vi "Register Create Test Node View.vi"(11 "Message Enqueuer in":refnum<class "Message Enqueuer.lvclass">) -> (3 "Message Enqueuer out":refnum<class "Message Enqueuer.lvclass">)   [LabVIEW 2013]
uses:
  <vilib>/ActorFramework/Message Enqueuer/Message Enqueuer.lvclass
  <vilib>/ActorFrameworkMVC/View Observer/Registration Message/Registration Message.lvclass
  <vilib>/ActorFrameworkMVC/View Observer/Data Message/Data Message.lvclass
  Models/Create Test Node Model Messages/Register Initialize Create Test Node Msg/Register Initialize Create Test Node Msg.lvclass
  Models/Create Test Node Model Messages/Register Set Create Test Node Key Focus Msg/Register Set Create Test Node Key Focus Msg.lvclass
  Views/Create Test Node View Messages/Conceret Initialize Create Test Node Msg/Conceret Initialize Create Test Node Msg.lvclass
  Views/Create Test Node View Messages/Conceret Set Create Test Node Key Focus Msg/Conceret Set Create Test Node Key Focus Msg.lvclass
  Views/Create Test Node View Messages/Conceret Create Test Node List Msg/Conceret Create Test Node List Msg.lvclass
  Models/Create Test Node Model Messages/Register Create Test Node List Msg/Register Create Test Node List Msg.lvclass
  <vilib>/ActorFrameworkMVC/UI Controller Messages/Subscribe View to Model Msg/Subscribe View to Model Msg.lvclass/Subscribe View to Model Msg.ctl
  <vilib>/ActorFramework/Message Enqueuer/Message Enqueuer.lvclass/Message Enqueuer.ctl
  <vilib>/ActorFramework/Message Enqueuer/Enqueue.vi
  <vilib>/ActorFramework/Message Priority Queue/Priority Enqueue.vi
  <vilib>/ActorFrameworkMVC/UI Controller Messages/Subscribe View to Model Msg/Subscribe View to Model Msg.lvclass
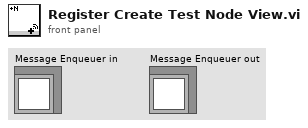
[diagram p1: front panel]
types:
  T1 = cluster{"Registration Message":string, "Data Message":string}[]
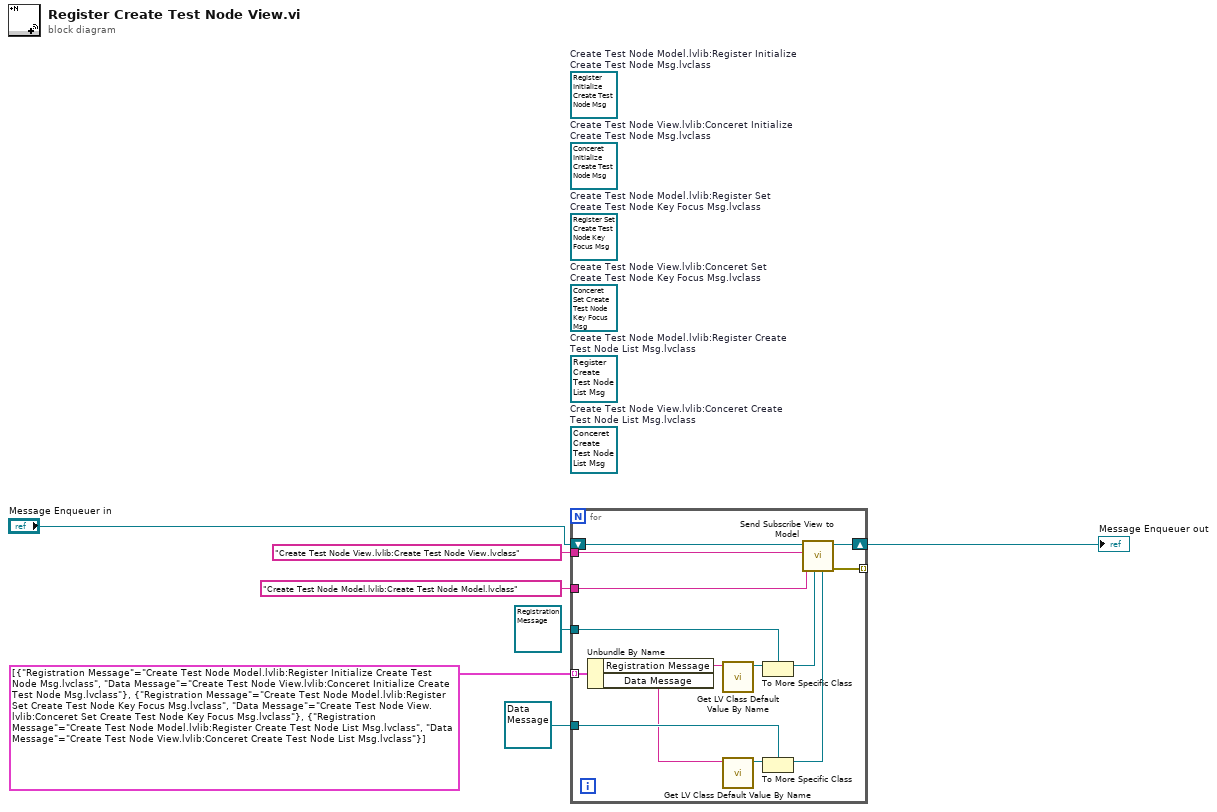
[diagram p0: block diagram]
diagram:
  (unwired) refnum<class "Register Create Test Node List Msg.lvclass"> refnum  # Create Test Node Model.lvlib:Register Create Test Node List Msg.lvclass
  (unwired) refnum<class "Conceret Create Test Node List Msg.lvclass"> refnum  # Create Test Node View.lvlib:Conceret Create Test Node List Msg.lvclass
  (unwired) refnum<class "Conceret Set Create Test Node Key Focus Msg.lvclass"> refnum  # Create Test Node View.lvlib:Conceret Set Create Test Node Key Focus Msg.lvclass
  (unwired) refnum<class "Conceret Initialize Create Test Node Msg.lvclass"> refnum  # Create Test Node View.lvlib:Conceret Initialize Create Test Node Msg.lvclass
  (unwired) refnum<class "Register Set Create Test Node Key Focus Msg.lvclass"> refnum  # Create Test Node Model.lvlib:Register Set Create Test Node Key Focus Msg.lvclass
  (unwired) refnum<class "Register Initialize Create Test Node Msg.lvclass"> refnum  # Create Test Node Model.lvlib:Register Initialize Create Test Node Msg.lvclass
  n1 = for {
    tunnel: "Create Test Node View.lvlib:Create Test Node View.lvclass" ("View Name") -> [w20]
    tunnel: "Create Test Node Model.lvlib:Create Test Node Model.lvclass" ("Model Name") -> [w19]
    shift-right: [w18] -> w6
    shift-left: "Message Enqueuer in" -> [w21]
    tunnel: refnum<class "Registration Message.lvclass"> refnum ("Registration Message") -> [w15]
    tunnel: refnum<class "Data Message.lvclass"> refnum ("Data Message") -> [w14]
    tunnel: T1 [{"Registration Message"="Create Test Node Model.lvlib:Register Initialize Create Test Node Msg.lvclass", "Data Message"="Create Test Node View.lvlib:Conceret Initialize Create Test Node Msg.lvclass"}, {"Registration Message"="Create Test Node Model.lvlib:Register Set Create Test Node Key Focus Msg.lvclass", "Data Message"="Create Test Node View.lvlib:Conceret Set Create Test Node Key Focus Msg.lvclass"}, {"Registration Message"="Create Test Node Model.lvlib:Register Create Test Node List Msg.lvclass", "Data Message"="Create Test Node View.lvlib:Conceret Create Test Node List Msg.lvclass"}] -> [w13] mode=indexing
    tunnel: [w8] -> _ mode=indexing
    n2 = Unbundle By Name(w13) -> ("Registration Message"=w10:string, "Data Message"=w9:string)
    n3 = call <vilib>:"Get LV Class Default Value By Name.vi"("class name"=w10) -> ("object"=w17:refnum<class>)  [unwired: 9 in, 1 out]
    n4 = call <vilib>:"Get LV Class Default Value By Name.vi"("class name"=w9) -> ("object"=w16:refnum<class>)  [unwired: 9 in, 1 out]
    n5 = To More Specific Class(target class=w15, reference=w17) -> (specific class reference=w12:refnum<class "Registration Message.lvclass">)  [unwired: 1 in, 1 out]
    n6 = To More Specific Class(target class=w14, reference=w16) -> (specific class reference=w11:refnum<class "Data Message.lvclass">)  [unwired: 1 in, 1 out]
    n7 = call <vilib>:"Send Subscribe View to Model.vi"("Data Message"=w11, "Registration Message"=w12, "Model Name"=w19, "View Name"=w20, "Message Enqueuer"=w21) -> ("error out"=w8:errorcluster, "Message Enqueuer out"=w18:refnum<class "Message Enqueuer.lvclass">)  [unwired: 5 in]
  }
  "Message Enqueuer out" <- w6
